vi "Start BuildWorker.vi"(8 "error in (no error)":errorcluster, 9 "Show":bool=TRUE, 10 "Port":i32=4545, 11 "BuildWorker Basics in":refnum<class "BuildWorker Basics.lvclass">) -> (0 "error out":errorcluster, 3 "BuildWorker Basics out":refnum<class "BuildWorker Basics.lvclass">)   [LabVIEW 2017, in "BuildWorker Controller.lvlib" / "BuildWorker Basics.lvclass"]
uses:
  BuildWorker Basics.lvclass
  Volumes/Data/Users/benji667/Git/BuildFarm/BuildWorker/Classes/BuildWorker/BuildWorker.lvclass
  BuildWorker/BuildWorker.lvclass/BuildWorker.ctl
  BuildWorker Basics.lvclass/BuildWorker Basics.ctl
  BuildWorker/Read Path.vi
  <vilib>/ActorFramework/Message Enqueuer/Message Enqueuer.lvclass
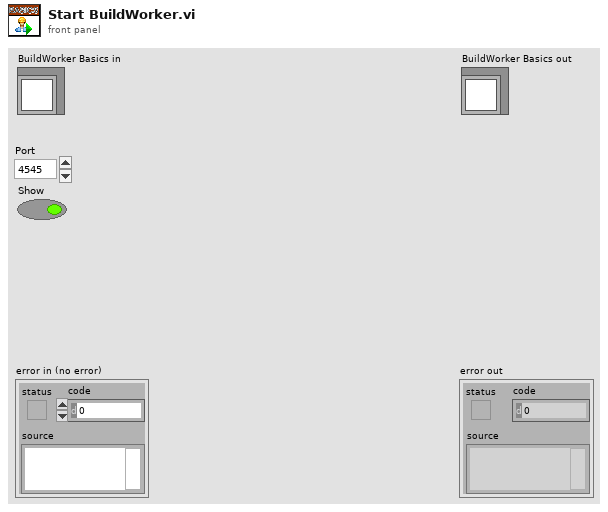
[diagram p1: front panel]
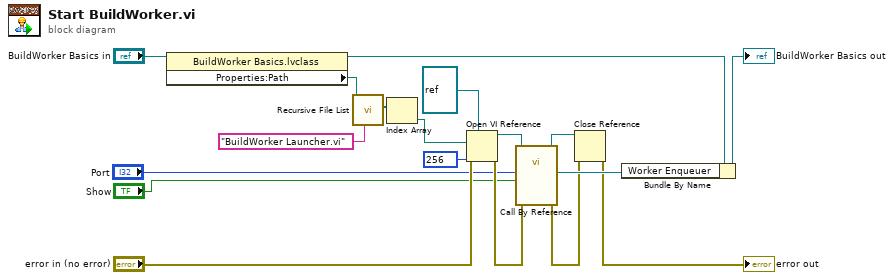
[diagram p0: block diagram]
diagram:
  n1 = property class="BuildWorker Basics.lvclass"(reference="BuildWorker Basics in") -> (reference out=w2:refnum<class "BuildWorker Basics.lvclass">, "Properties:Path"=w1:path)  [unwired: 1 in, 1 out]
  n2 = call <vilib>:"Recursive File List.vi"("pattern"="BuildWorker Launcher.vi" ("VI Path"), "Folder Path"=w1) -> ("All Files in Dir"=w4:path[])  [unwired: 5 in, 4 out]
  n3 = Index Array(array=w4) -> (element=w3:path)  [unwired: 1 in]
  n4 = Open VI Reference(type specifier VI Refnum (for type only)=refnum<vi> refnum, vi path=w3, options=256, error in (no error)="error in (no error)") -> (vi reference=w13:refnum<vi>, error out=w12:errorcluster)  [unwired: 2 in]
  n5 = call-by-ref "?"(reference=w13, error in=w12, "Show"="Show", "Port"="Port") -> (reference out=w8:refnum<vi>, error out=w7:errorcluster, "Worker Enqueuer"=w9:refnum<class "Message Enqueuer.lvclass">)  [unwired: 9 in]
  n6 = Close Reference(reference=w8, error in (no error)=w7) -> (error out=→"error out":errorcluster)
  n7 = Bundle By Name(cluster=w2, "Worker Enqueuer"=w9) -> (→"BuildWorker Basics out":refnum<class "BuildWorker Basics.lvclass">)
